vi "Fetch Accessor Type.vi"(8 "Error in":errorcluster caption="Error in (no error)", 11 "VI in":refnum<vi>) -> (0 "Error out":errorcluster, 3 "VI Type Ext":T1)   [LabVIEW 2023, in "VIDoc Parsing.lvlib"]
uses:
  VIDoc Parsing.lvlib
  TypeDefs/VI Type Extended Enum.ctl
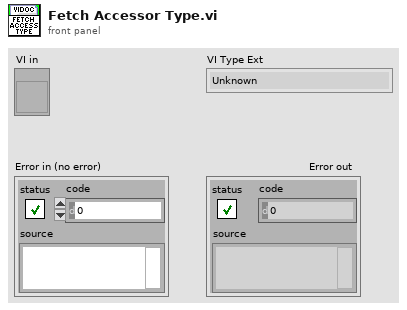
[diagram p1: front panel]
types:
  T1 = typedef "VIDoc Parsing.lvlib/VI Type Extended Enum.ctl" = enum16{"Unknown", "Class Method", "Class Accessor Get", "Class Accessor Set", "Class Control", "Library Method", "Library Control", "VI", "Control"}
  T2 = typedef "LVRectTypeDef.ctl" = cluster{"Left":i16, "Top":i16, "Right":i16, "Bottom":i16}
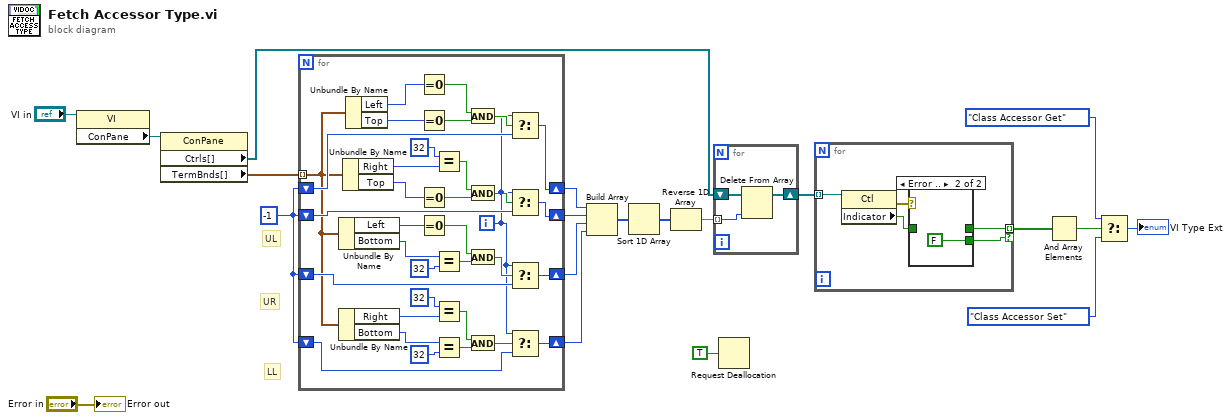
[diagram p0: block diagram]
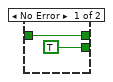
[diagram p2: hidden frame]
diagram:
  w12 = -1
  # "LL"
  # "UR"
  # "UL"
  n1 = property class="VI"(reference="VI in") -> ("ConPane"=w6:refnum<vi>)  [unwired: 1 in, 2 out]
  n2 = property class="ConPane"(reference=w6) -> ("Ctrls[]"=w14:refnum<vi>[], "TermBnds[]"=w13:T2[])  [unwired: 1 in, 2 out]
  n3 = for {
    tunnel: w13 -> [w21] mode=indexing
    shift-right: [w48] -> w11
    shift-left: w12 -> [w49]
    shift-right: [w40] -> w10
    shift-left: w12 -> [w41]
    shift-right: [w32] -> w9
    shift-left: w12 -> [w33]
    shift-right: [w22] -> w8
    shift-left: w12 -> [w23]
    i -> [w24]
    n4 = Unbundle By Name(w21) -> ("Left"=w38:i16, "Bottom"=w36:i16)
    n5 = Unbundle By Name(w21) -> ("Right"=w27:i16, "Bottom"=w30:i16)
    n6 = Unbundle By Name(w21) -> ("Right"=w45:i16, "Top"=w46:i16)
    n7 = Unbundle By Name(w21) -> ("Left"=w54:i16, "Top"=w53:i16)
    n8 = Equal To 0?(x=w54) -> (x = 0?=w52:bool)
    n9 = Equal To 0?(x=w53) -> (x = 0?=w51:bool)
    n10 = Equal To 0?(x=w46) -> (x = 0?=w47:bool)
    n11 = Equal To 0?(x=w38) -> (x = 0?=w39:bool)
    n12 = Equal?(x=i16 32, y=w45) -> (x = y?=w43:bool)
    n13 = Equal?(x=w36, y=i16 32 ("x")) -> (x = y?=w37:bool)
    n14 = Equal?(x=i16 32, y=w27) -> (x = y?=w26:bool)
    n15 = Equal?(x=w30, y=i16 32 ("x")) -> (x = y?=w29:bool)
    n16 = And(x=w52, y=w51) -> (x .and. y?=w50:bool)
    n17 = And(x=w43, y=w47) -> (x .and. y?=w42:bool)
    n18 = And(x=w39, y=w37) -> (x .and. y?=w34:bool)
    n19 = And(x=w26, y=w29) -> (x .and. y?=w25:bool)
    n20 = Select(t=w24, s=w50, f=w49) -> (s? t:f=w48:i32)
    n21 = Select(t=w24, s=w42, f=w41) -> (s? t:f=w40:i32)
    n22 = Select(t=w24, s=w34, f=w33) -> (s? t:f=w32:i32)
    n23 = Select(t=w24, s=w25, f=w23) -> (s? t:f=w22:i32)
  }
  n24 = Build Array(w11, w10, w9, w8) -> (w15:i32[])
  n25 = Sort 1D Array(array=w15) -> (sorted array=w16:i32[])
  n26 = Reverse 1D Array(array=w16) -> (reversed array=w17:i32[])
  n27 = for {
    shift-right: [w56] -> w18
    shift-left: w14 -> [w57]
    tunnel: w17 -> [w55] mode=indexing
    n28 = Delete From Array(array=w57, index=w55) -> (array with subset deleted=w56:refnum<vi>[])  [unwired: 1 in, 1 out]
  }
  n29 = Request Deallocation(TRUE ("flag")) -> ()
  n30 = for {
    tunnel: w18 -> [w62] mode=indexing
    tunnel: [w59] -> w19 mode=indexing if=w58
    n31 = property class="Ctl"(reference=w62) -> (error out=w61:errorcluster, "Indicator"=w60:bool)  [unwired: 1 in, 1 out]
    n32 = case shown="Error .." w61 {
      tunnel: w60 -> [w64 _]
      tunnel: [w64 _] -> w59
      tunnel: [TRUE FALSE] -> w58
      frame No Error {
      }
      frame Error {
      }
    }
  }
  n33 = And Array Elements(Boolean array=w19) -> (logical AND=w20:bool)
  n34 = Select(t=VI_Type_Extended_Enum."Class Accessor Get", s=w20, f=VI_Type_Extended_Enum."Class Accessor Set") -> (s? t:f=→"VI Type Ext":T1)
  "Error out" <- "Error in"
